vi "Create.vi"(10 "Log Status":T1) -> (3 "Log Status Value out":refnum<class "Log Status Value.lvclass">)   [LabVIEW 2020, in "VolatusData.lvlib" / "Log Status Value.lvclass"]
uses:
  Log Status Value.lvclass
  Log Status.ctl
  Logging State.ctl
  Log Status Value.lvclass/Log Status Value.ctl
  VolatusData.lvlib
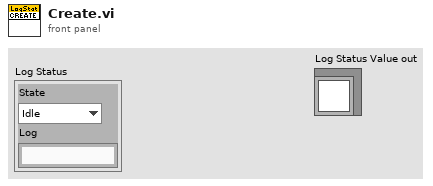
[diagram p1: front panel]
types:
  T1 = typedef "VolatusData.lvlib/Log Status.ctl" = cluster{"State":T2, "Log":string}
  T2 = typedef "VolatusData.lvlib/Logging State.ctl" = enum16{"Idle", "Starting", "Logging", "Stopping"}
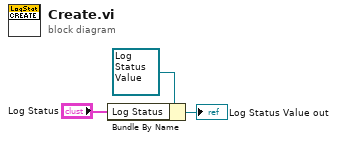
[diagram p0: block diagram]
diagram:
  n1 = Bundle By Name(cluster=refnum<class "Log Status Value.lvclass"> refnum ("Log Status Value out"), "Log Status"="Log Status") -> (→"Log Status Value out":refnum<class "Log Status Value.lvclass">)
